vi "v0.2_limpiar_enc_http.vi"(8 "error in":errorcluster, 11 "mbed.lvclass IN":refnum<class "mbed.lvclass">) -> (0 "error out":errorcluster, 3 "mbed.lvclass OUT":refnum<class "mbed.lvclass">)   [LabVIEW 2011]
doc: "<B>Servo ON</B>\n\nEncender/Apagar el servomotor utilizando una variable boolena"
uses:
  C:/mbed/Transport Mechanisms/mbed/mbed.lvclass
  C:/mbed/mbed Interface/RPCFunction/RPCFunction.lvclass
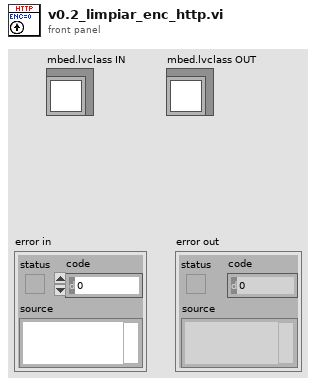
[diagram p1: front panel]
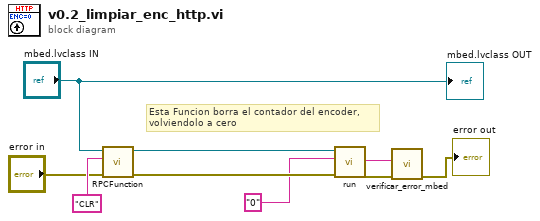
[diagram p0: block diagram]
diagram:
  # "Esta Funcion borra el contador del encoder, \nvolviendolo a cero"
  n1 = call "RPCFunction.vi"("error in (no error)"="error in", "Existing Obj Name"="CLR", "mbed_LVLibrary.lvlib:mbed.lvclass"="mbed.lvclass IN") -> ("error out"=w4:errorcluster, "mbed_LVLibrary.lvlib:Packet.lvclass 2"=w8:refnum<class "RPCFunction.lvclass">)  [unwired: 6 in, 1 out]
  n2 = call "run.vi"("error in (no error)"=w4, "Input"="0", "Packet in"=w8) -> ("error out"=w6:errorcluster, "Output"=w2:string)  [unwired: 6 in, 1 out]
  n3 = call "verificar_error_mbed.vi"("error in (no error)"=w6, "desde_mbed"=w2) -> ("error out"=→"error out":errorcluster)  [unwired: 8 in, 1 out]
  "mbed.lvclass OUT" <- "mbed.lvclass IN"
